vi "Wait for Device Response.vi"(8 "error in (no error)":errorcluster, 10 "Delay Time (s) (0.1s)":dbl=0.3, 11 "heater_parent in":refnum<class "heater_parent.lvclass">) -> (0 "error out":errorcluster, 3 "heater_parent out":refnum<class "heater_parent.lvclass">)   [LabVIEW 2020, in "polar_bear_plus_drivers.lvlib" / "heater_parent.lvclass"]
doc: "This VI should be inserted before a \"Read from Instrument\" VI that immediately follows a \"Write to Instrument\" VI. Based on the VI provided by VICI to test communications with flow actuators, we also wait for 300 ms between a Write and the corresponding Read."
uses:
  <instrlib>/RxnRover/Driver Polar Bear Plus/heater_parent/heater_parent.lvclass
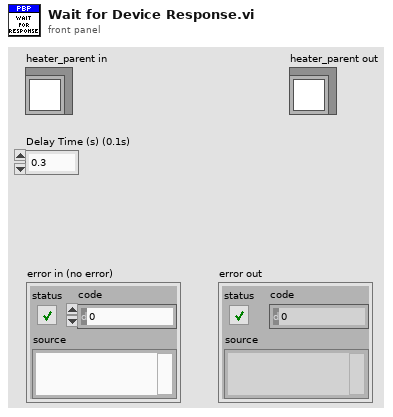
[diagram p1: front panel]
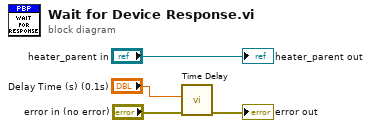
[diagram p0: block diagram]
diagram:
  n1 = call "Time Delay"("error in (no error)"="error in (no error)", "Delay Time (s)"="Delay Time (s) (0.1s)") -> ("error out"=→"error out":errorcluster)  [unwired: 9 in]
  "heater_parent out" <- "heater_parent in"
